vi "Write Program List.vi"(8 "error in (no error)":errorcluster, 10 "Program List.lvclass":refnum<class "Program List.lvclass">, 11 "Program Interface in":refnum<class "Program Interface.lvclass">) -> (0 "error out":errorcluster, 3 "Program Interface out":refnum<class "Program Interface.lvclass">)   [LabVIEW 2019, in "Program Interface.lvclass"]
uses:
  Program Interface.lvclass
  Program List.lvclass
  Program Interface.lvclass/Program Interface.ctl
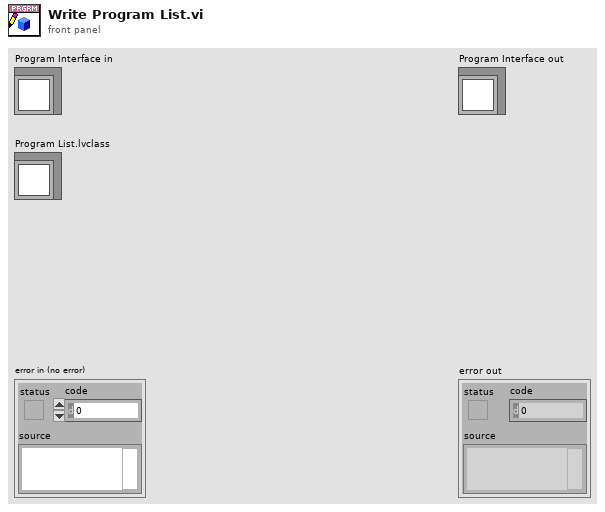
[diagram p1: front panel]
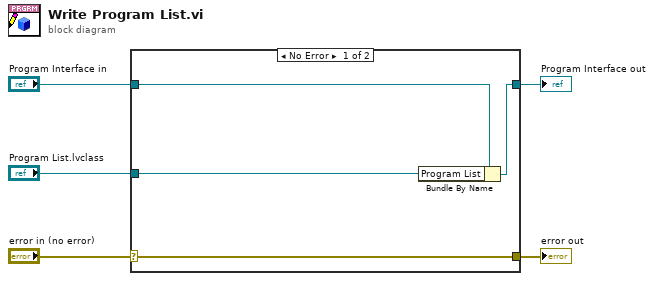
[diagram p0: block diagram]
diagram:
  n1 = case shown="No Error" "error in (no error)" {
    selector: "error in (no error)" -> [w9 w10]
    tunnel: [w9 w10] -> w4
    tunnel: [w7 w11] -> w2
    tunnel: "Program Interface in" -> [w8 w11]
    tunnel: "Program List.lvclass" -> [w6 _]
    frame No Error {
      n2 = Bundle By Name(cluster=w8, "Program List"=w6) -> (w7:refnum<class "Program Interface.lvclass">)
    }
    frame Error {
    }
  }
  "error out" <- w4
  "Program Interface out" <- w2
